vi "One or More.vi"(8 "error in (no error)":errorcluster, 11 "Mock in":refnum<class "Mock.lvclass">) -> (0 "error out":errorcluster, 3 "Mock out":refnum<class "Mock.lvclass">)   [LabVIEW 2020, in "One or More.lvclass"]
uses:
  One Of/One or More.lvclass
  Mock/Mock.lvclass
  C:/git/astemes-lmock/sandbox/Expectation/Expectation.lvclass
  One Of/One or More.lvclass/One or More.ctl
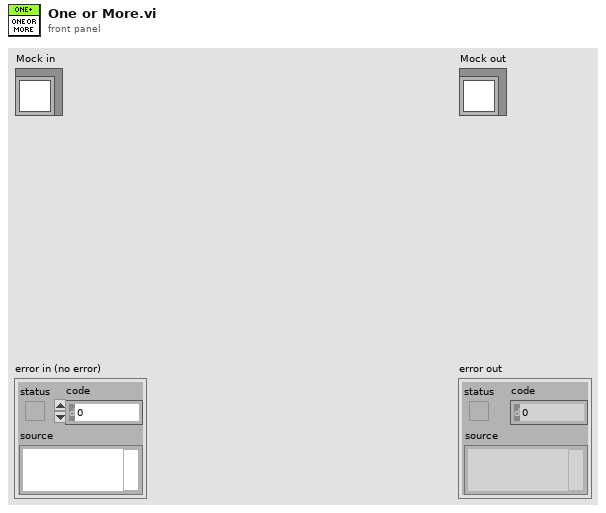
[diagram p1: front panel]
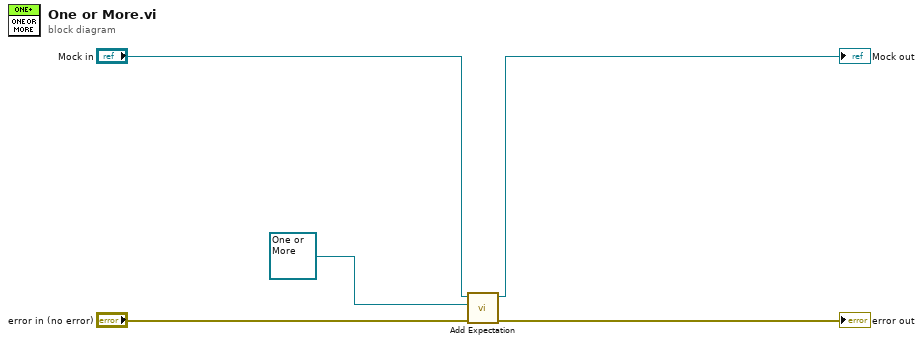
[diagram p0: block diagram]
diagram:
  n1 = call "Add Expectation.vi"("error in (no error)"="error in (no error)", "Expectations"=refnum<class "One or More.lvclass"> refnum ("One Of.lvclass"), "Mock in"="Mock in") -> ("error out"=→"error out":errorcluster, "Mock out"=→"Mock out":refnum<class "Mock.lvclass">)  [unwired: 7 in]
